vi "Custom Probe Demo.vi"() -> ()   [LabVIEW 2017]
uses:
  Classes/Person/Person.lvclass
panel:
  in  "Date Of Birth":timestamp=timestamp(2508824327.797493 s since 1904-01-01) format="%<%x>T"
  in  "Last Name":string="R"
  in  "First Name":string="Benjamin"
  out "Person out":refnum<class "Person.lvclass">
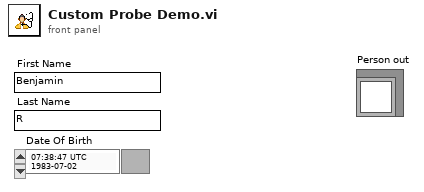
[diagram p1: front panel]
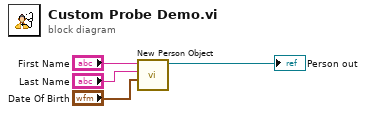
[diagram p0: block diagram]
diagram:
  n1 = call "New Person Object.vi"("Date Of Birth"="Date Of Birth", "Last Name"="Last Name", "First Name"="First Name") -> ("Person out"=→"Person out":refnum<class "Person.lvclass">)  [unwired: 7 in, 1 out]
